vi "Scan for Devices on System.vi"(8 "error in (no error)":errorcluster) -> (0 "error out":errorcluster, 2 "Changed?":bool, 3 "Resources out":refnum<k20>[](array[refnum]))   [LabVIEW 2017, in "Controller Actor.lvlib" / "Controller.lvclass"]
uses:
  Controller.lvclass
  <vilib>/nisyscfg/Filter Mode.ctl
  <vilib>/nisyscfg/nisyscfg.lvlib
  <resource>/objmgr/niMIDebugSession.rc
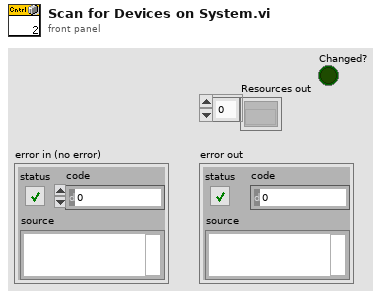
[diagram p1: front panel]
types:
  T1 = typedef "nisyscfg.lvlib/Filter Mode.ctl" = i32
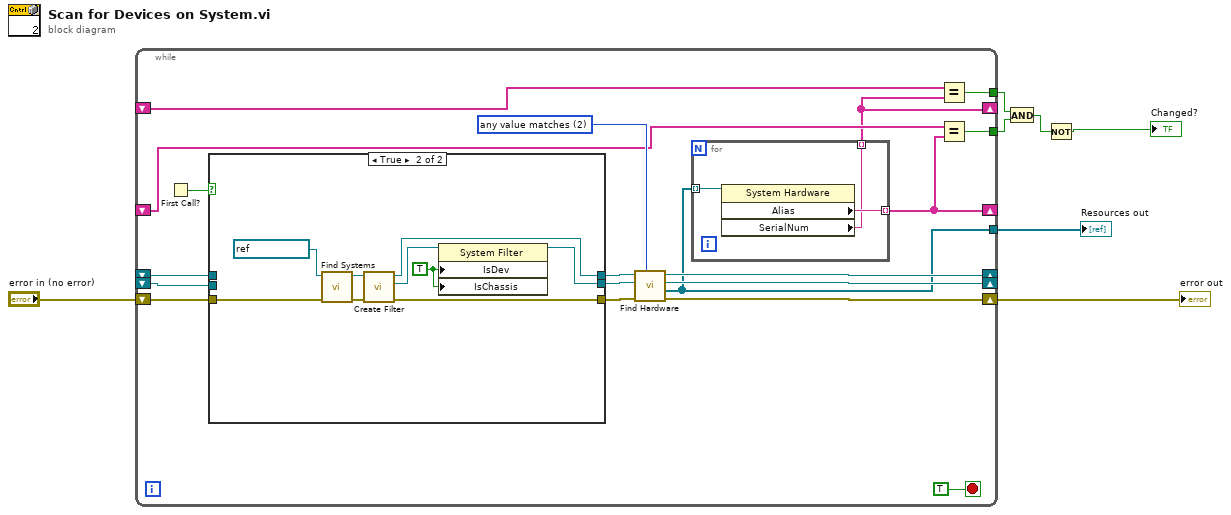
[diagram p0: block diagram]
diagram:
  n1 = while {
    tunnel: [w14] -> w7
    shift-right: [w25] -> w5
    shift-left: "error in (no error)" -> [w26]
    shift-right: [w24] -> _
    shift-left: _ -> [w16]
    shift-right: [w17] -> _
    shift-left: _ -> [w15]
    shift-right: [w13] -> _
    shift-left: _ -> [w12]
    tunnel: [w11] -> w2
    tunnel: [w10] -> w3
    shift-right: [w9] -> _
    shift-left: _ -> [w8]
    stop <- TRUE stop-if-true
    w20 = T1 2 items=["all values match"=1, "any value matches"=2, "values do not match"=3, "all properties exist"=4] ("Filter Mode (all values match)")
    n2 = First Call?() -> (First Call?: T/F=w18:bool)
    n3 = case shown="True" w18 {
      tunnel: w26 -> [w30 w41]
      tunnel: [w32 w39] -> w23
      tunnel: [w30 w36] -> w22
      tunnel: [w31 w35] -> w21
      tunnel: w16 -> [w32 _]
      tunnel: w15 -> [w31 _]
      frame False {
      }
      frame True {
        w40 = TRUE ("Is Device")
        n4 = call <vilib>:"Find Systems.vi"("error in (no error)"=w41, "Session in (localhost)"=refnum<k21> "localhost") -> ("error out"=w37:errorcluster, "Session out"=w38:refnum<k21>)  [unwired: 7 in, 1 out]
        n5 = call <vilib>:"Create Filter.vi"("error in (no error)"=w37, "Session in"=w38) -> ("error out"=w36:errorcluster, "Filter out"=w34:refnum<k20>, "Session out"=w39:refnum<k21>)  [unwired: 7 in]
        n6 = property class="System Filter"(reference=w34, "IsDev"=w40, "IsChassis"=w40) -> (reference out=w35:refnum<k20>)  [unwired: 1 in, 1 out]
      }
    }
    n7 = call <vilib>:"Find Hardware.vi"("Filter Mode (all values match)"=w20, "error in (no error)"=w22, "Filter in"=w21, "Session in"=w23) -> ("error out"=w25:errorcluster, "Resources out"=w14:refnum<k20>[], "Filter out"=w17:refnum<k20>, "Session out"=w24:refnum<k21>)  [unwired: 4 in]
    n8 = for {
      tunnel: w14 -> [w29] mode=indexing
      tunnel: [w28] -> w13 mode=indexing
      tunnel: [w27] -> w9 mode=indexing
      n9 = property class="System Hardware"(reference=w29) -> ("Alias"=w28:string, "SerialNum"=w27:string)  [unwired: 1 in, 2 out]
    }
    n10 = Equal?(x=w8, y=w9) -> (x = y?=w10:bool)
    n11 = Equal?(x=w12, y=w13) -> (x = y?=w11:bool)
  }
  "Resources out" <- w7
  "error out" <- w5
  n12 = And(x=w3, y=w2) -> (x .and. y?=w1:bool)
  n13 = Not(x=w1) -> (.not. x?=→"Changed?":bool)
